vi "YAFFooter_CastUIEvent.vi"(11 "UIEvent":T2) -> (1 "Data":variant, 2 "ApplicationGUIOut":refnum<class "YAFFooter.lvclass">, 3 "UiEventNames":T1)   [LabVIEW 2021, in "YAFFooter.lvlib" / "YAFFooter.lvclass"]
uses:
  YAFFooter.lvclass
  YAFFooter.lvclass/YAFFooter.ctl
  YAFFooter_UiCallBackEvents.ctl
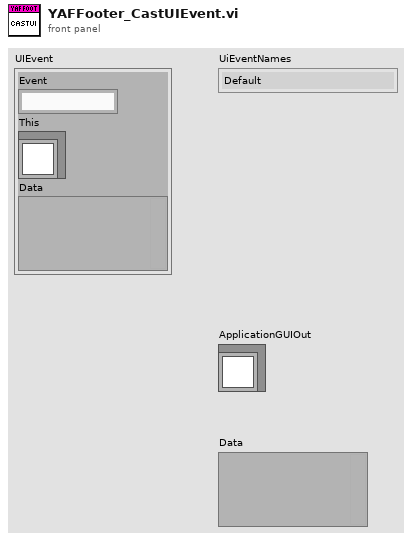
[diagram p1: front panel]
types:
  T1 = typedef "YAFFooter.lvlib/YAFFooter.lvclass/YAFFooter_UiCallBackEvents.ctl" = enum16{"Default", "PersistentDataUpdated"}
  T2 = cluster{"Event":string, "This":refnum<class>, "Data":variant}
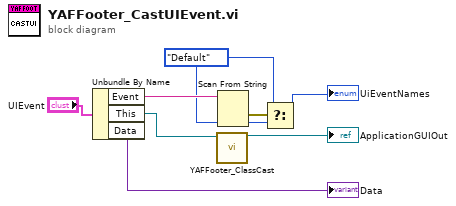
[diagram p0: block diagram]
diagram:
  w2 = YAFFooter_UiCallBackEvents."Default" ("UiEventNames")
  n1 = Unbundle By Name("UIEvent") -> ("Event"=w6:string, "This"=w5:refnum<class>, "Data"=→"Data":variant)
  n2 = call "YAFFooter_ClassCast.vi"("YAFFooter:YAFFooter in"=w5) -> ("YAFFooter:YAFFooter out"=→"ApplicationGUIOut":refnum<class "YAFFooter.lvclass">)  [unwired: 10 in]
  n3 = Scan From String(input string=w6, default 1=w2) -> (error out=w9:errorcluster, output 1=w4:T1)  [unwired: 3 in, 2 out]
  n4 = Select(t=w2, s=w9, f=w4) -> (s? t:f=→"UiEventNames":T1)
